vi "Disable buttons.vi"(8 "error in (no error)":errorcluster, 10 "Disabled":T1(ring), 11 "Array":refnum<vi>[](array[refnum])) -> (0 "error out":errorcluster)   [LabVIEW 2020]
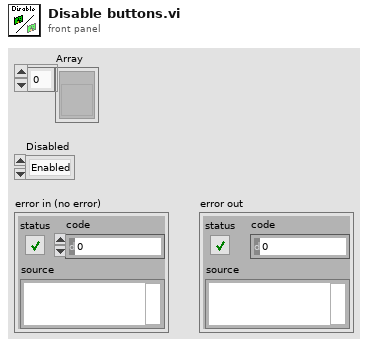
[diagram p1: front panel]
types:
  T1 = enum8{"Enabled", "Disabled", "Disabled and Grayed Out"}
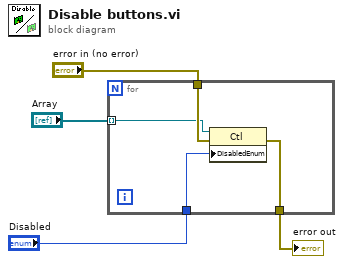
[diagram p0: block diagram]
diagram:
  n1 = for {
    tunnel: "Disabled" -> [w8]
    tunnel: [w7] -> w2
    tunnel: "Array" -> [w5] mode=indexing
    tunnel: "error in (no error)" -> [w6]
    n2 = property class="Ctl"(reference=w5, error in=w6, "DisabledEnum"=w8) -> (error out=w7:errorcluster)  [unwired: 1 out]
  }
  "error out" <- w2
